vi "claw work 4.vi"   [LabVIEW 2010, in "ClawBot.lvrbt"]
uses:
  ClawBot.lvrbt
  <vilib>/NXT/Block Support/NXT_InputPort.ctl
  <vilib>/NXT/Subs/MotorOutput.ctl
  <vilib>/NXT/Dual Mode Library/Motors/Rotation.vi
  <vilib>/NXT/Dual Mode Library/Sensors/Sonar_cm.vi
  <vilib>/NXT/Dual Mode Library/Motors/MotorOn.vi
  <vilib>/NXT/Dual Mode Library/Motors/MotorBrake.vi
types:
  T1 = typedef "NXT_InputPort.ctl" = u8
  T2 = typedef "MotorOutput.ctl" = u8
  T3 = typedef "LVHSConnector.ctl" = cluster{"Hardware":string, "Flattened String":string}
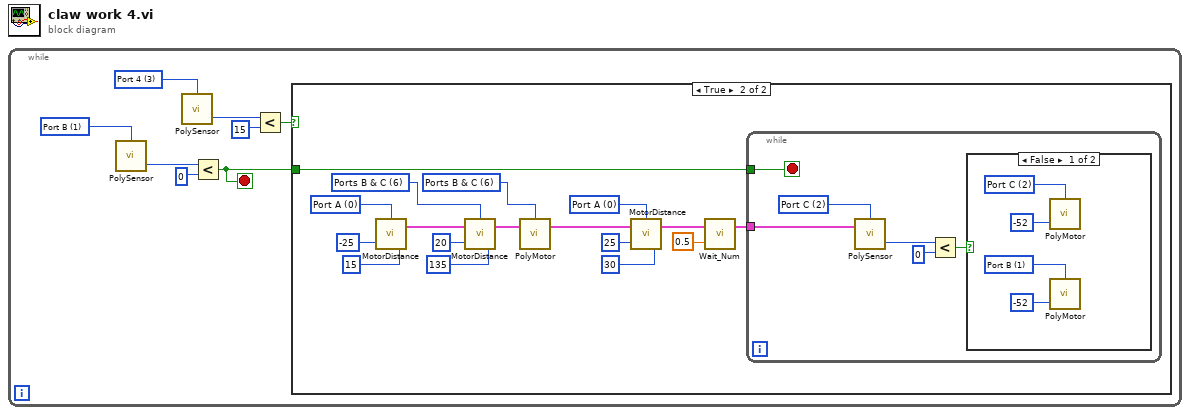
[diagram p0: block diagram]
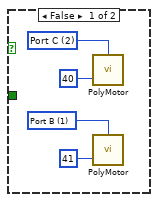
[diagram p2: hidden frame]
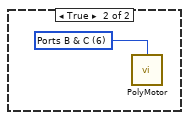
[diagram p3: hidden frame]
diagram:
  n1 = while {
    stop <- w1 stop-if-true
    w4 = u8 1 items=["Port A", "Port B", "Port C"] ("Port (Port A)")
    w7 = T1 3 items=["Port 1", "Port 2", "Port 3", "Port 4"] ("Port (Port 4)")
    n2 = call-poly <vilib>:"PolySensor.vi"("Port (Port A)"=w4) -> ("Angle of Rotation"=w5:i32)  [unwired: 2 in, 1 out]
    n3 = call-poly <vilib>:"PolySensor.vi"("Port (Port 4)"=w7) -> ("Distance (cm)"=w3:i16)  [unwired: 2 in, 1 out]
    n4 = Less?(x=w5, y=i16 0 ("Distance (cm)")) -> (x < y?=w1:bool)
    n5 = Less?(x=w3, y=i16 15 ("Distance (cm)")) -> (x < y?=w2:bool)
    n6 = case shown="True" w2 {
      tunnel: w1 -> [_ w13]
      frame False {
        w10 = T2 2 items=["Port A"=0, "Port B"=1, "Port C"=2, "Ports A & B"=4, "Ports A & C"=5, "Ports B & C"=6, "All Ports"=3] ("Output Port (All Ports)")
        w12 = T2 1 items=["Port A"=0, "Port B"=1, "Port C"=2, "Ports A & B"=4, "Ports A & C"=5, "Ports B & C"=6, "All Ports"=3] ("Output Port (All Ports)")
        n7 = call-poly <vilib>:"PolyMotor.vi"("Power (75)"=40, "Output Port (All Ports)"=w10) -> ()  [unwired: 2 in, 1 out]
        n8 = call-poly <vilib>:"PolyMotor.vi"("Power (75)"=41, "Output Port (All Ports)"=w12) -> ()  [unwired: 2 in, 1 out]
      }
      frame True {
        w19 = T2 6 items=["Port A"=0, "Port B"=1, "Port C"=2, "Ports A & B"=4, "Ports A & C"=5, "Ports B & C"=6, "All Ports"=3] ("Output Port (All Ports)")
        w23 = T2 0 items=["Port A"=0, "Port B"=1, "Port C"=2, "Ports A & B"=4, "Ports A & C"=5, "Ports B & C"=6, "All Ports"=3] ("Output Port (All Ports)")
        w26 = T2 0 items=["Port A"=0, "Port B"=1, "Port C"=2, "Ports A & B"=4, "Ports A & C"=5, "Ports B & C"=6, "All Ports"=3] ("Output Port (All Ports)")
        w29 = T2 6 items=["Port A"=0, "Port B"=1, "Port C"=2, "Ports A & B"=4, "Ports A & C"=5, "Ports B & C"=6, "All Ports"=3] ("Port (All Ports)")
        n9 = call <vilib>:"MotorDistance.vi"("Power (75)"=-25, "Angle of Rotation (360)"=15, "Output Port (All Ports)"=w26) -> ("NXT"=w18:T3)  [unwired: 1 in]
        n10 = call <vilib>:"MotorDistance.vi"("Power (75)"=20, "Angle of Rotation (360)"=135, "NXT"=w18, "Output Port (All Ports)"=w19) -> ("NXT"=w17:T3)
        n11 = call-poly <vilib>:"PolyMotor.vi"("NXT"=w17, "Port (All Ports)"=w29) -> ("NXT"=w14:T3)  [unwired: 2 in]
        n12 = call <vilib>:"MotorDistance.vi"("Power (75)"=25, "Angle of Rotation (360)"=30, "NXT"=w14, "Output Port (All Ports)"=w23) -> ("NXT"=w21:T3)
        n13 = call <vilib>:"Wait_Num.vi"("Time (1 sec)"=sgl 0.5, "NXT"=w21) -> ("NXT"=w15:T3)  [unwired: 2 in]
        n14 = while {
          tunnel: w15 -> [w35]
          tunnel: w13 -> [w30]
          stop <- w30 stop-if-true
          w32 = u8 2 items=["Port A", "Port B", "Port C"] ("Port (Port A)")
          n15 = call-poly <vilib>:"PolySensor.vi"("NXT"=w35, "Port (Port A)"=w32) -> ("Angle of Rotation"=w33:i32)  [unwired: 1 in, 1 out]
          n16 = Less?(x=w33, y=i16 0 ("Distance (cm)")) -> (x < y?=w31:bool)
          n17 = case shown="False" w31 {
            frame False {
              w37 = T2 2 items=["Port A"=0, "Port B"=1, "Port C"=2, "Ports A & B"=4, "Ports A & C"=5, "Ports B & C"=6, "All Ports"=3] ("Output Port (All Ports)")
              w39 = T2 1 items=["Port A"=0, "Port B"=1, "Port C"=2, "Ports A & B"=4, "Ports A & C"=5, "Ports B & C"=6, "All Ports"=3] ("Output Port (All Ports)")
              n18 = call-poly <vilib>:"PolyMotor.vi"("Power (75)"=-52, "Output Port (All Ports)"=w37) -> ()  [unwired: 2 in, 1 out]
              n19 = call-poly <vilib>:"PolyMotor.vi"("Power (75)"=-52, "Output Port (All Ports)"=w39) -> ()  [unwired: 2 in, 1 out]
            }
            frame True {
              w40 = T2 6 items=["Port A"=0, "Port B"=1, "Port C"=2, "Ports A & B"=4, "Ports A & C"=5, "Ports B & C"=6, "All Ports"=3] ("Output Port (All Ports)")
              n20 = call-poly <vilib>:"PolyMotor.vi"("Port (All Ports)"=w40) -> ()  [unwired: 3 in, 1 out]
            }
          }
        }
      }
    }
  }
